vi "Get Active Targets.vi"(8 "error in (no error)":errorcluster, 10 "Minutes":i32, 11 "UI Data in":T1) -> (0 "error out":errorcluster, 1 "Cool Setpoint (°F)":dbl, 2 "Heat Setpoint (°F)":dbl, 3 "UI Data out":T1)   [LabVIEW 2026]
uses:
  controls/UI Data.ctl
  controls/User Settings.ctl
  controls/Schedule Interval.ctl
  controls/System Status Displays.ctl
  controls/Manual Override.ctl
  controls/Global Settings.ctl
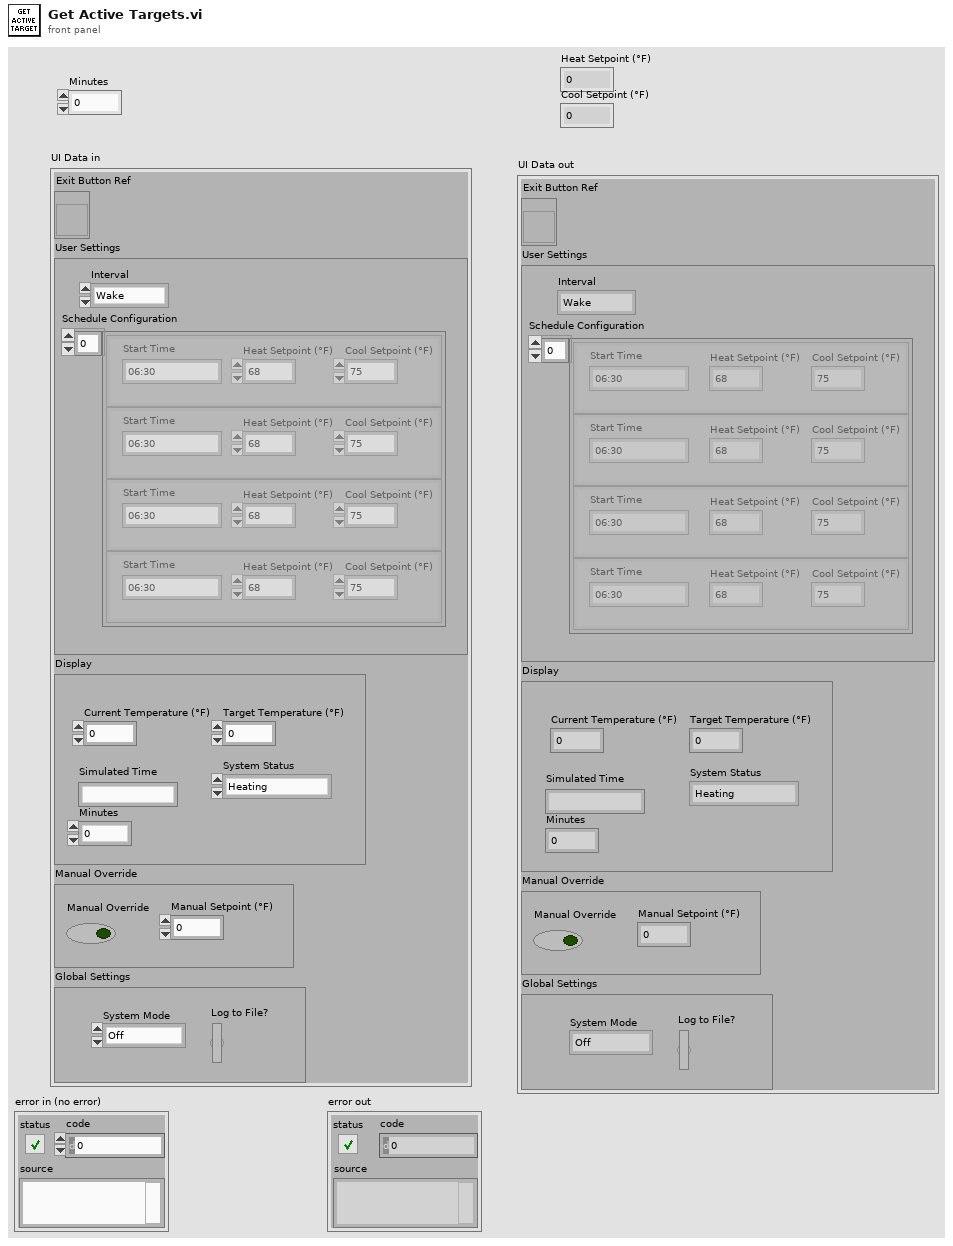
[diagram p1: front panel]
types:
  T1 = typedef "UI Data.ctl" = cluster{"Exit Button Ref":refnum<vi>, "User Settings":T2, "Display":T4, "Manual Override":T5, "Global Settings":T6}
  T2 = typedef "User Settings.ctl" = cluster{"Schedule Configuration":cluster{"Start Time":string, "Heat Setpoint (°F)":dbl, "Cool Setpoint (°F)":dbl}[], "Interval":T3}
  T3 = typedef "Schedule Interval.ctl" = enum16{"Wake", "Leave", "Return", "Sleep"}
  T4 = typedef "System Status Displays.ctl" = cluster{"Current Temperature (°F)":dbl, "Target Temperature (°F)":dbl, "System Status":enum16{"Heating", "Cooling", "Idle"}, "Simulated Time":string, "Minutes":i16}
  T5 = typedef "Manual Override.ctl" = cluster{"Manual Override":bool, "Manual Setpoint (°F)":dbl}
  T6 = typedef "Global Settings.ctl" = cluster{"System Mode":enum16{"Off", "Cool", "Auto", "Heat"}, "Log to File?":bool}
  T7 = cluster{"Start Time":string, "Heat Setpoint (°F)":dbl, "Cool Setpoint (°F)":dbl}[]
  T8 = cluster{"Start Time":string, "Heat Setpoint (°F)":dbl, "Cool Setpoint (°F)":dbl}
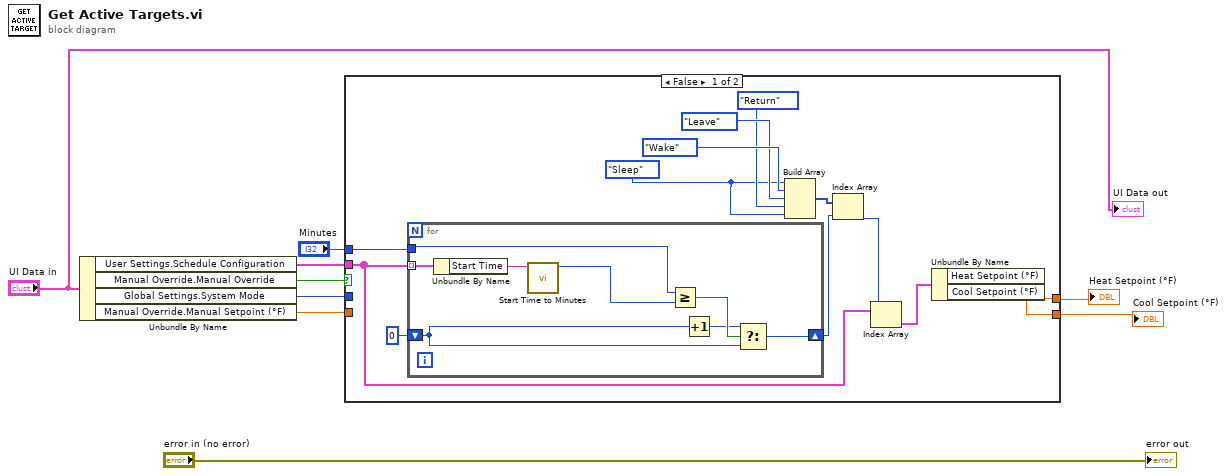
[diagram p0: block diagram]
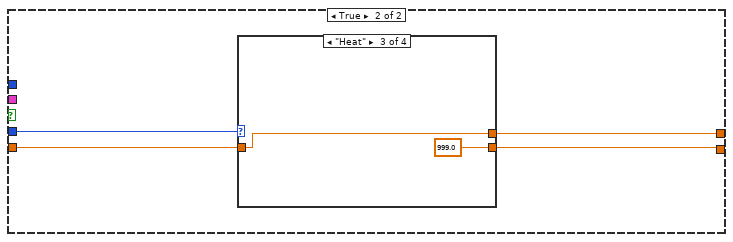
[diagram p2: hidden frame]
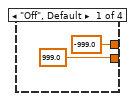
[diagram p3: hidden frame]
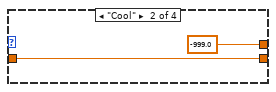
[diagram p4: hidden frame]
diagram:
  n1 = Unbundle By Name("UI Data in") -> ("User Settings.Schedule Configuration"=w8:T7, "Manual Override.Manual Override"=w5:bool, "Global Settings.System Mode"=w4:enum16{"Off", "Cool", "Auto", "Heat"}, "Manual Override.Manual Setpoint (°F)"=w3:dbl)
  n2 = case shown="False" w5 {
    tunnel: w8 -> [w15 _]
    tunnel: [w13 w31] -> w7
    tunnel: [w12 w32] -> w6
    tunnel: w4 -> [_ w34]
    tunnel: w3 -> [_ w33]
    tunnel: "Minutes" -> [w11 _]
    frame False {
      w10 = Schedule_Interval."Sleep"
      n3 = for {
        tunnel: w15 -> [w30] mode=indexing
        shift-right: [w26] -> w17
        shift-left: 0 -> [w24]
        tunnel: w11 -> [w23]
        n4 = Unbundle By Name(w30) -> ("Start Time"=w29:string)
        n5 = call "Start Time to Minutes.vi"("Start Time"=w29) -> ("Minutes"=w28:i32)  [unwired: 9 in, 1 out]
        n6 = Greater Or Equal?(x=w23, y=w28) -> (x >= y?=w27:bool)
        n7 = Increment(x=w24) -> (x+1=w25:i32)
        n8 = Select(t=w25, s=w27, f=w24) -> (s? t:f=w26:i32)
      }
      n9 = Build Array(w10, Schedule_Interval."Wake", Schedule_Interval."Leave", Schedule_Interval."Return", w10) -> (w19:T3[])
      n10 = Index Array(array=w19, index=w17) -> (element=w16:T3)
      n11 = Index Array(array=w15, index=w16) -> (element=w14:T8)
      n12 = Unbundle By Name(w14) -> ("Heat Setpoint (°F)"=w13:dbl, "Cool Setpoint (°F)"=w12:dbl)
    }
    frame True {
      n13 = case shown="\"Heat\"" w34 {
        tunnel: w33 -> [_ w38 w39 w41]
        tunnel: [999.0 ("Manual Setpoint (°F)") w38 999.0 ("Manual Setpoint (°F)") w41] -> w32
        tunnel: [-999.0 ("Manual Setpoint (°F)") -999.0 ("Manual Setpoint (°F)") w39 w41] -> w31
        frame "Off", Default {
        }
        frame "Cool" {
        }
        frame "Heat" {
        }
        frame "Auto" {
        }
      }
    }
  }
  "Heat Setpoint (°F)" <- w7
  "Cool Setpoint (°F)" <- w6
  "error out" <- "error in (no error)"
  "UI Data out" <- "UI Data in"
